vi "Non-Broadcast Call.vi"(7 "Emergency Stop? (F)":bool, 8 "error in (no error)":errorcluster, 11 "API-Reference in":refnum<k1>) -> (0 "error out":errorcluster, 3 "API-Reference out":refnum<k1>)   [LabVIEW 2018, in "Copy of Actor.lvclass"]
uses:
  Copy of Actor.lvclass
  Stop.ctl
  Launched.ctl
  Event-References.ctl
  Stopped.ctl
  API-Data.ctl
  Some Request.ctl
  Some Response.ctl
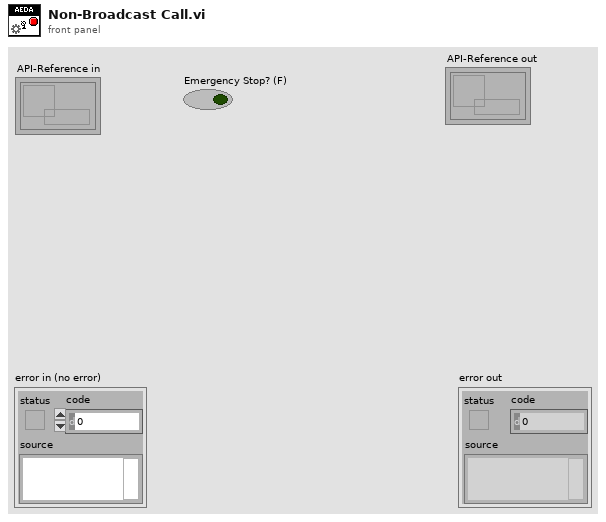
[diagram p1: front panel]
types:
  T1 = typedef "Copy of Actor.lvclass/API-Data.ctl" = cluster{"Launch":refnum<notifier>, "Stopped":refnum<user-event>, "Actor-Events":T2, "Stopped Registration":refnum<event-registration>}
  T2 = typedef "Copy of Actor.lvclass/Event-References.ctl" = cluster{"Stop":refnum<user-event>, "Launched":refnum<user-event>, "Some Request":refnum<user-event>}
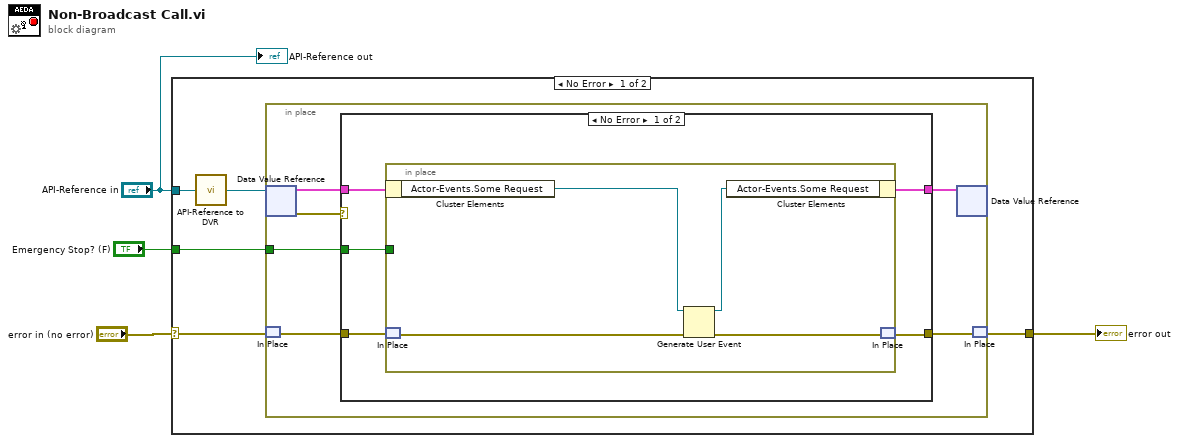
[diagram p0: block diagram]
diagram:
  n1 = case shown="No Error" "error in (no error)" {
    selector: "error in (no error)" -> [w9 w27]
    tunnel: [w8 w27] -> w2
    tunnel: "API-Reference in" -> [w5 _]
    tunnel: "Emergency Stop? (F)" -> [w7 _]
    frame No Error {
      n2 = call "API-Reference to DVR.vi"("API-Reference in"=w5) -> ("Data Value Reference out"=w6:refnum<data-value>)
      n3 = in-place {
        in-place-border: w7 -> [w10]
        n4 = in-place-dvr #1(w6) -> (w14:T1, w15:errorcluster)
        n5 = in-place-match #2(w9) -> (w12:errorcluster)
        n6 = case shown="No Error" w15 {
          selector: w15 -> [_ w26]
          tunnel: w14 -> [w18 w25]
          tunnel: [w16 w25] -> w13
          tunnel: w12 -> [w20 _]
          tunnel: [w19 w26] -> w11
          tunnel: w10 -> [w17 _]
          frame No Error {
            n7 = in-place {
              in-place-border: w17 -> [_]
              n8 = in-place-cluster #3(w18) -> ("Actor-Events.Some Request"=w23:refnum<user-event>)
              n9 = in-place-match #4(w20) -> (w24:errorcluster)
              n10 = Generate User Event(user event=w23, error in=w24) -> (user event out=w22:refnum<user-event>, error out=w21:errorcluster)  [unwired: 2 in]
              n11 = in-place-cluster #3("Actor-Events.Some Request"=w22) -> (w16:T1)
              n12 = in-place-match #4(w21) -> (w19:errorcluster)
            }
          }
          frame Error {
          }
        }
        n13 = in-place-dvr #1(w13) -> ()  [unwired: 2 out]
        n14 = in-place-match #2(w11) -> (w8:errorcluster)
      }
    }
    frame Error {
    }
  }
  "error out" <- w2
  "API-Reference out" <- "API-Reference in"
